vi "GetPAQ_TAGs.vi"(8 "error in (no error)":errorcluster, 11 "FAMM in":refnum<class "FAMM.lvclass">) -> (0 "error out":errorcluster, 2 "PAQ_TAGs":string[](array[string]), 3 "FAMM out":refnum<class "FAMM.lvclass">)   [LabVIEW 2014, in "FAMM.lvclass"]
uses:
  FAMM.lvclass
  FAMM.lvclass/FAMM.ctl
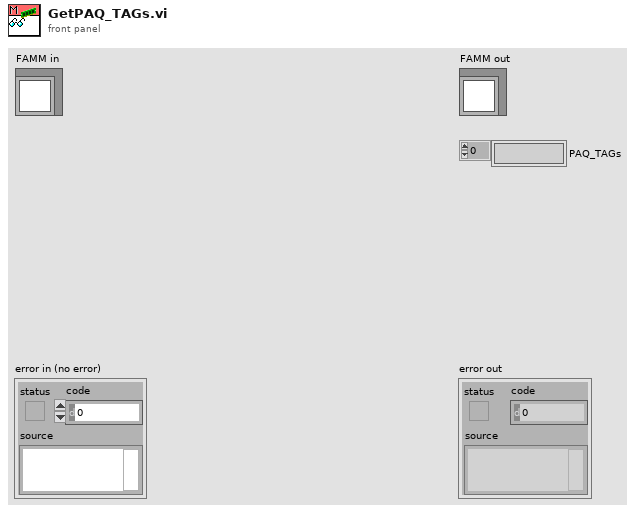
[diagram p1: front panel]
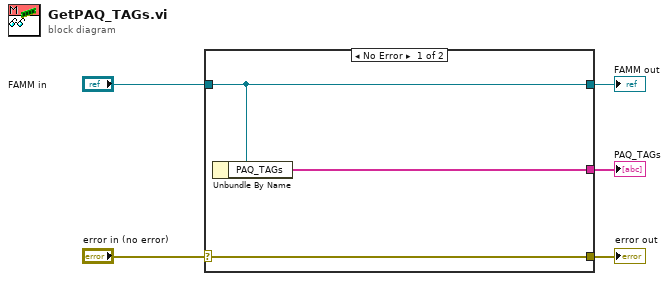
[diagram p0: block diagram]
diagram:
  n1 = case shown="No Error" "error in (no error)" {
    selector: "error in (no error)" -> [w8 w9]
    tunnel: [w8 w9] -> w4
    tunnel: [w7 w10] -> w2
    tunnel: "FAMM in" -> [w7 w10]
    tunnel: [w6 _] -> w1
    frame No Error {
      n2 = Unbundle By Name(w7) -> ("PAQ_TAGs"=w6:string[])
    }
    frame Error {
    }
  }
  "error out" <- w4
  "FAMM out" <- w2
  "PAQ_TAGs" <- w1
